vi "Get previous month.vi"() -> (0 "Year":i32, 3 "Month (1-12)":i32)   [LabVIEW 2015]
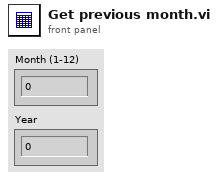
[diagram p1: front panel]
types:
  T1 = typedef "LVDateTimeRec.ctl" = cluster{"fractional second":dbl, "second":i32, "minute":i32, "hour":i32, "day of month":i32, "month":i32, "year":i32, "day of week":i32, "day of year":i32, "DST":i32}
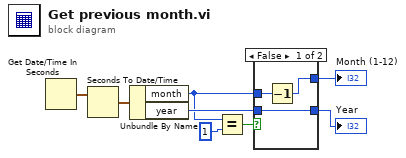
[diagram p0: block diagram]
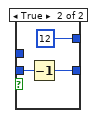
[diagram p2: hidden frame]
diagram:
  n1 = Get Date/Time In Seconds() -> (seconds since 1Jan1904=w8:timestamp)
  n2 = Seconds To Date/Time(time stamp (now)=w8) -> (date time rec=w6:T1)  [unwired: 1 in]
  n3 = Unbundle By Name(w6) -> ("month"=w1:i32, "year"=w4:i32)
  n4 = Equal?(x=w1, y=1) -> (x = y?=w5:bool)
  n5 = case shown="False" w5 {
    tunnel: w4 -> [w11 w14]
    tunnel: [w11 w13] -> w3
    tunnel: [w10 12] -> w2
    tunnel: w1 -> [w9 _]
    frame False {
      n6 = Decrement(x=w9) -> (x-1=w10:i32)
    }
    frame True {
      n7 = Decrement(x=w14) -> (x-1=w13:i32)
    }
  }
  "Year" <- w3
  "Month (1-12)" <- w2
